vi "se3e2.vi"() -> ()   [LabVIEW 2013]
panel:
  out "Average":cluster{"number: 0 to 1":dbl, dbl}(graph)
  in  "?":bool
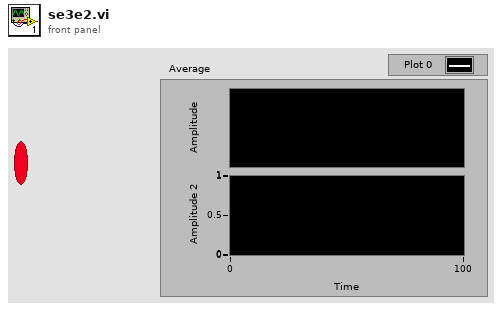
[diagram p1: front panel]
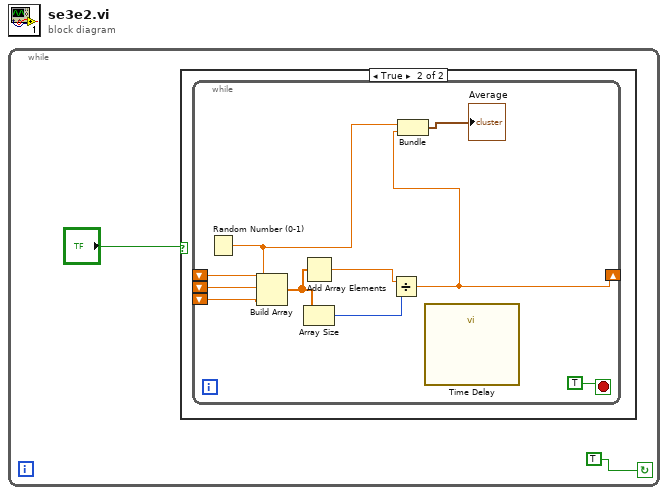
[diagram p0: block diagram]
diagram:
  n1 = while {
    stop <- TRUE continue-if-true
    n2 = case shown="True" "?" {
      frame False {
      }
      frame True {
        n3 = while {
          shift-right: [w4] -> _
          shift-left: _ -> [w12]
          shift-left: _ -> [w10]
          shift-left: _ -> [w11]
          stop <- TRUE stop-if-true
          n4 = Random Number (0-1)() -> (number: 0 to 1=w5:dbl)
          n5 = Build Array(w5, w12, w11, w10) -> (w9:dbl[])
          n6 = Add Array Elements(numeric array=w9) -> (sum=w8:dbl)
          n7 = Array Size(array=w9) -> (size(s)=w7:i32)
          n8 = Divide(x=w8, y=w7) -> (x/y=w4:dbl)
          n9 = Bundle("number: 0 to 1"=w5, w4) -> (→"Average":cluster{"number: 0 to 1":dbl, dbl})  [unwired: 1 in]
          n10 = call "Time Delay"() -> ()  [unwired: 11 in, 1 out]
        }
      }
    }
  }
